vi "Create PPL Build Spec.vi"(8 "error in (no error)":errorcluster, 10 "measurement plug-in name":string, 11 "project refnum":refnum<vi>) -> (0 "error out":errorcluster, 2 "measurement UI built path":path, 3 "project ref out":refnum<vi>)   [LabVIEW 2021, in "MeasurementService Editor.lvlib"]
uses:
  MeasurementService Editor.lvlib
  <vilib>/AppBuilder/AB_API/PPL/NI_AB_API_PPL.lvclass
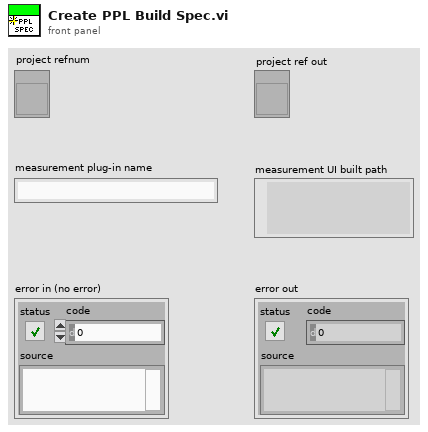
[diagram p1: front panel]
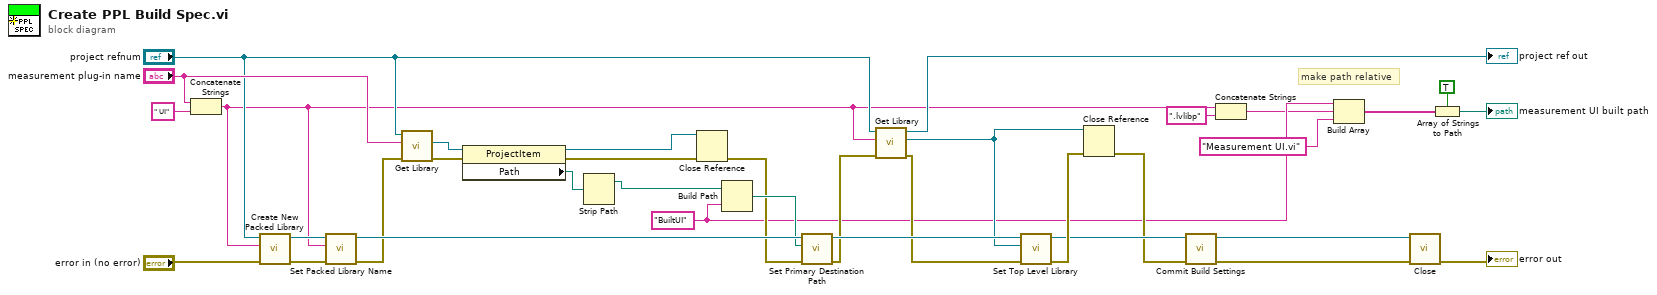
[diagram p0: block diagram]
diagram:
  w8 = "BuiltUI" ("y")
  # "make path relative"
  n1 = Concatenate Strings("measurement plug-in name", " UI" ("string")) -> (w6:string)
  n2 = call <vilib>:"Create New Packed Library.vi"("error in (no error)"="error in (no error)", "Build specification name"=w6, "Project Refnum"="project refnum") -> ("error out"=w34:errorcluster, "PPL out"=w33:refnum<class "NI_AB_API_PPL.lvclass">)  [unwired: 7 in]
  n3 = call-dynamic "Set Packed Library Name.vi"("error in (no error)"=w34, "Packed library name"=w6, "PPL in"=w33) -> ("error out"=w27:errorcluster, "PPL out"=w29:refnum<class "NI_AB_API_PPL.lvclass">)  [unwired: 7 in]
  n4 = call "Get Library.vi"("error in (no error)"=w27, "library name"="measurement plug-in name", "project ref"="project refnum") -> ("error out"=w25:errorcluster, "library item"=w26:refnum<vi>)  [unwired: 5 in, 2 out]
  n5 = property class="ProjectItem"(reference=w26, error in=w25) -> (reference out=w22:refnum<vi>, error out=w23:errorcluster, "Path"=w13:path)
  n6 = Strip Path(path=w13) -> (stripped path=w12:path)  [unwired: 1 out]
  n7 = Close Reference(reference=w22, error in (no error)=w23) -> (error out=w21:errorcluster)
  n8 = Build Path(base path=w12, name or relative path=w8) -> (appended path=w24:path)
  n9 = call-dynamic "Set Primary Destination Path.vi"("error in (no error)"=w21, "Destination path"=w24, "Build in"=w29) -> ("error out"=w20:errorcluster, "Build out"=w30:refnum<class "NI_AB_API_PPL.lvclass">)  [unwired: 7 in]
  n10 = call "Get Library.vi"("error in (no error)"=w20, "library name"=w6, "project ref"="project refnum") -> ("error out"=w18:errorcluster, "library item"=w16:refnum<vi>, "project ref out"=→"project ref out":refnum<vi>)  [unwired: 5 in, 1 out]
  n11 = call-dynamic "Set Top Level Library.vi"("error in (no error)"=w18, "ProjectItem Refnum"=w16, "PPL in"=w30) -> ("error out"=w17:errorcluster, "PPL out"=w15:refnum<class "NI_AB_API_PPL.lvclass">)  [unwired: 7 in]
  n12 = Close Reference(reference=w16, error in (no error)=w17) -> (error out=w14:errorcluster)
  n13 = call-dynamic "Commit Build Settings.vi"("error in (no error)"=w14, "PPL in"=w15) -> ("error out"=w2:errorcluster, "PPL out"=w3:refnum<class "NI_AB_API_PPL.lvclass">)  [unwired: 8 in]
  n14 = Concatenate Strings(w6, ".lvlibp" ("string")) -> (w7:string)
  n15 = Build Array(w8, w7, "Measurement UI.vi" ("element")) -> (w1:string[])
  n16 = call-dynamic "Close.vi"("error in (no error)"=w2, "DLL in"=w3) -> ("error out"=→"error out":errorcluster)  [unwired: 9 in]
  n17 = Array of Strings to Path(0:w1, 1:TRUE ("relative")) -> (2:→"measurement UI built path":path)
